vi "calibrationSpectrometer_getEvent_TimeOut.vi"(8 "error in (no error)":errorcluster, 11 "logevent_TimeOut_Ctl":T1) -> (0 "error out":errorcluster, 2 "function return":i32, 3 "logevent_TimeOut_Ctl out":T1)   [LabVIEW 2016, in "SALLV_calibrationSpectrometer.lvlib"]
doc: "int calibrationSpectrometer_shm_getEvent_TimeOutLV(calibrationSpectrometer_logevent_TimeOutLV *logevent_TimeOut_Ctl );"
uses:
  SALLV_calibrationSpectrometer.lvlib
  DataTypes/logevent_TimeOut.ctl
  SALLV_calibrationSpectrometer.so
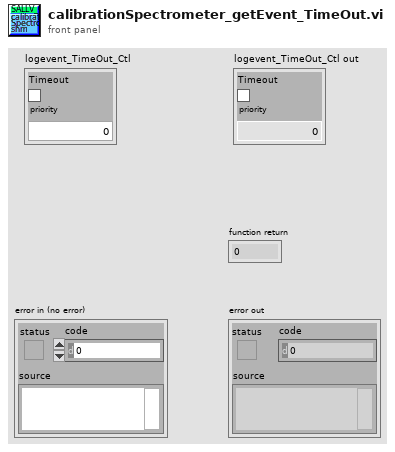
[diagram p1: front panel]
types:
  T1 = typedef "SALLV_calibrationSpectrometer.lvlib/logevent_TimeOut.ctl" = cluster{"Timeout":bool, "priority":i32}
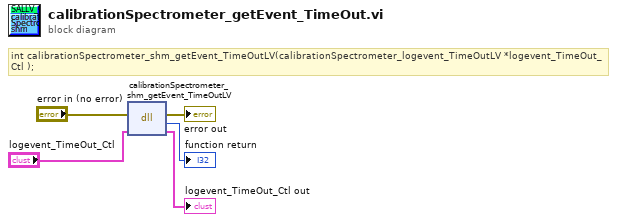
[diagram p0: block diagram]
diagram:
  # "int calibrationSpectrometer_shm_getEvent_TimeOutLV(calibrationSpectrometer_logevent_TimeOutLV *logevent_TimeOut_Ctl );"
  n1 = dll-call lib="home/harini/TCS/sallv_sedspectrometer/SALLV_calibrationSpectrometer.*" fn="calibrationSpectrometer_shm_getEvent_TimeOutLV"(error in="error in (no error)", "logevent_TimeOut_Ctl"="logevent_TimeOut_Ctl") -> (error out=→"error out":errorcluster, →"function return":i32, "logevent_TimeOut_Ctl"=→"logevent_TimeOut_Ctl out":T1)  [unwired: 2 in, 1 out]
